vi "Look for EOF keyword.vi"(7 "EOF text":string="ENDOFFILE", 8 "file string":string, 9 "Complete record = T":bool, 10 "HEADER string start index":i32, 11 "sweep record string":string) -> (0 "Stop Loop, EOC":bool, 1 "Complete record = T":bool, 2 "Key word start index":i32, 3 "sweep record string out":string, 4 "ENDOFFILE":bool)   [LabVIEW 2018]
doc: "Because the rcord detection string match looks for two consecutive key words:\nHEADER,\nit won't work for the very last record.\nTherefore, I added a second keyword at the end of every file,\nENDOFFILE\n\nI think this wiould be faster than other solutions like counting rows in every reocord.\nI think this would be more scaleable than using the keyword 6000000000 (6GHz in the last row of every record) becasue that wouldn't work for other frequency bands.\n-cc BSoft"
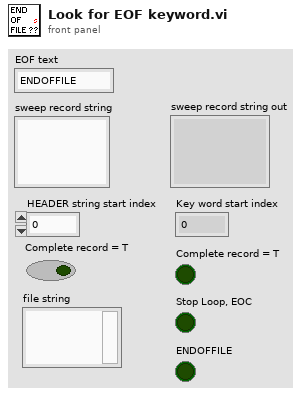
[diagram p1: front panel]
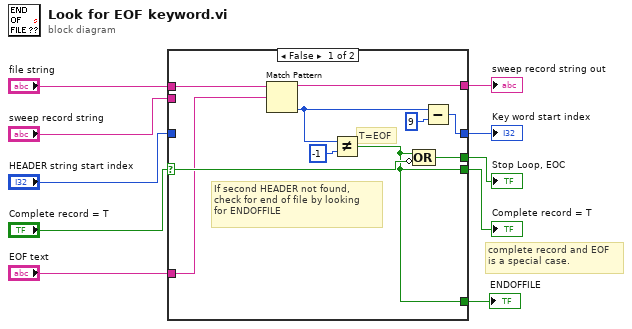
[diagram p0: block diagram]
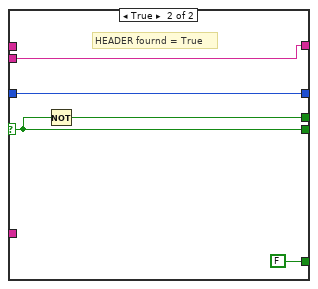
[diagram p2: hidden frame]
diagram:
  # "complete record and EOF\nis a special case."
  n1 = case shown="False" "Complete record = T" {
    selector: "Complete record = T" -> [w14 w23]
    tunnel: "file string" -> [w17 _]
    tunnel: [w16 w25] -> w9
    tunnel: [w12 w23] -> w8
    tunnel: "HEADER string start index" -> [_ w25]
    tunnel: [w15 w24] -> w5
    tunnel: "sweep record string" -> [_ w24]
    tunnel: [w13 w22] -> w3
    tunnel: [w12 FALSE] -> w2
    tunnel: "EOF text" -> [w11 _]
    frame False {
      # "If second HEADER not found, \ncheck for end of file by looking \nfor ENDOFFILE"
      # "T=EOF"
      n2 = Match Pattern(string=w17, regular expression=w11) -> (before substring=w15:string, offset past match=w20:i32)  [unwired: 1 in, 2 out]
      n3 = Not Equal?(x=w20, y=-1) -> (x != y?=w12:bool)
      n4 = Compound Arithmetic op=OR(w12, invert w14) -> (w13:bool)
      n5 = Subtract(x=w20, y=9) -> (x-y=w16:i32)
    }
    frame True {
      # "HEADER fournd = True"
      n6 = Not(x=w23) -> (.not. x?=w22:bool)
    }
  }
  "Key word start index" <- w9
  "Complete record = T" <- w8
  "sweep record string out" <- w5
  "Stop Loop, EOC" <- w3
  "ENDOFFILE" <- w2
